vi "Mult-Plex Switch POC.Async.vi"(10 "Parameters":variant, 11 "Process":refnum<class "Process.lvclass">) -> ()   [LabVIEW 2021, in "Software Multi-Plex Engine.lvlib"]
uses:
  Software Multi-Plex Engine.lvlib
  <vilib>/NI/NIVS Inline Async API/_VS Inline Async API/Process/Process.lvclass
  <vilib>/NI/NIVS Inline Async API/_VS Inline Async API/Process/Process.lvclass/Process.ctl
  Shared/Compiled.Settings.ctl
  <vilib>/NI/NIVS Inline Async API/_Data Access Engine/Access Type Classes/Read/Read.lvclass/Read.ctl
  <vilib>/NI/NIVS Inline Async API/_Data Access Engine/Access Type Classes/Write/Write.lvclass/Write.ctl
  <vilib>/NI/NIVS Inline Async API/_Data Access Engine/Data Access Engine/Methods/Read.Data.Detect.vi
  <vilib>/NI/NIVS Inline Async API/_Data Access Engine/Data Access Engine/Methods/Write.Data.vi
  <vilib>/NI/NIVS Inline Async API/_VS Inline Async API/Process/Data Member Access/Read Data Access.vi
  <vilib>/NI/NIVS Inline Async API/_VS Inline Async API/Error Handling Process/SubVIs/Error.ConvertArray.vi
  <vilib>/NI/NIVS Inline Async API/_Data Access Engine/Access Type Classes/Read/Read.ProcessData.Detect.vi
  <vilib>/NI/NIVS Inline Async API/_Data Access Engine/Access Type Classes/Write/Write.ProcessData.vi
  <vilib>/NI/NIVS Inline Async API/_Data Access Engine/Access Type Classes/Write/Write.Buffer.vi
  <vilib>/NI/NIVS Inline Async API/_Data Access Engine/Access Type Classes/Write/Write.Commit.vi
  <vilib>/NI/NIVS Inline Async API/_Data Access Engine/Data Access Engine/Methods/Read.Lookup.vi
  <vilib>/NI/NIVS Inline Async API/_Data Access Engine/Data Access Engine/Methods/Write.Lookup.vi
  <vilib>/NI/NIVS Inline Async API/_Data Access Engine/Data Access Engine/Data Access Engine.lvclass
  Shared/Software Multi-Plex Shared.lvlib
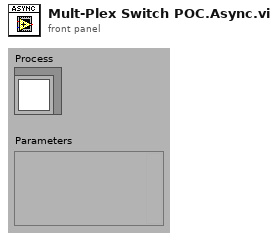
[diagram p1: front panel]
types:
  T1 = typedef "Software Multi-Plex Shared.lvlib/Compiled.Settings.ctl" = cluster{"Name":string, "Number of Channels":i32, "Inputs per Channel":i32, "Global Selector":bool}
  T2 = typedef "Data Access Engine.lvlib/Data Access Engine.lvclass/Read.DVR.ctl" = refnum<data-value>
  T3 = typedef "Data Access Engine.lvlib/Data Access Engine.lvclass/Write.DVR.ctl" = refnum<data-value>
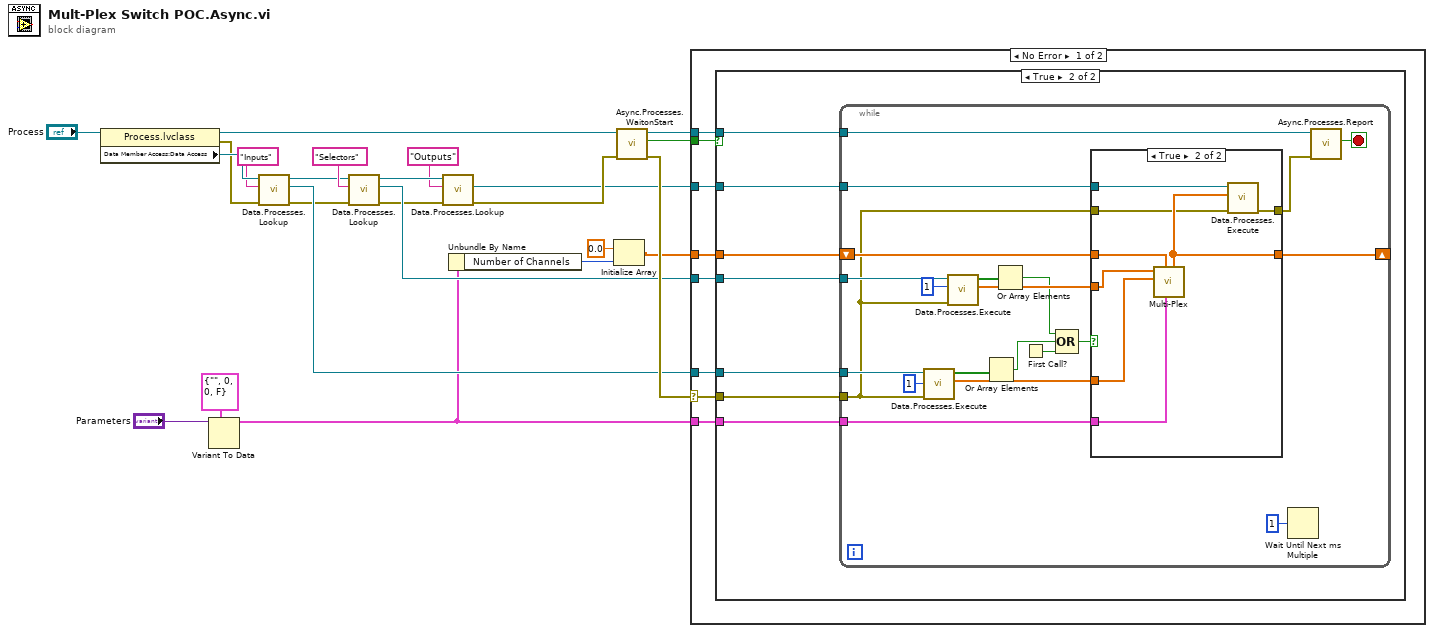
[diagram p0: block diagram]
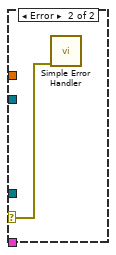
[diagram p4: hidden frame]
diagram:
  n1 = property class="Process.lvclass"(reference="Process") -> (reference out=w20:refnum<class "Process.lvclass">, error out=w13:errorcluster, "Data Member Access:Data Access"=w14:refnum<class "Data Access Engine.lvclass">)  [unwired: 1 in]
  n2 = Variant To Data(type=T1 {"Name"="", "Number of Channels"=0, "Inputs per Channel"=0, "Global Selector"=FALSE} ("Compiled.Settings"), Variant="Parameters") -> (data=w2:T1)  [unwired: 1 in, 1 out]
  n3 = call-poly <vilib>:"Data.Processes.Lookup.vi"("error in (no error)"=w13, "Name"="Inputs", "Data Access API in"=w14) -> ("error out"=w6:errorcluster, "Ref"=w12:T2, "Data Access API out"=w5:refnum<class "Data Access Engine.lvclass">)  [unwired: 5 in, 1 out]
  n4 = call-poly <vilib>:"Data.Processes.Lookup.vi"("error in (no error)"=w6, "Name"="Selectors", "Data Access API in"=w5) -> ("error out"=w9:errorcluster, "Ref"=w16:T2, "Data Access API out"=w19:refnum<class "Data Access Engine.lvclass">)  [unwired: 5 in, 1 out]
  n5 = call-poly <vilib>:"Data.Processes.Lookup.vi"("error in (no error)"=w9, "Name"="Outputs", "Data Access API in"=w19) -> ("error out"=w17:errorcluster, "Ref"=w15:T3)  [unwired: 5 in, 2 out]
  n6 = Unbundle By Name(w2) -> ("Number of Channels"=w1:i32)
  n7 = Initialize Array(0.0 ("element"), w1) -> (w3:dbl[])
  n8 = call <vilib>:"Async.Processes.WaitonStart.vi"("error in (no error)"=w17, "Process"=w20) -> ("error out"=w22:errorcluster, "Execute"=w24:bool, "Process out"=w23:refnum<class "Process.lvclass">)  [unwired: 7 in]
  n9 = case shown="No Error" w22 {
    selector: w22 -> [w30 w71]
    tunnel: w24 -> [w32 _]
    tunnel: w23 -> [w31 _]
    tunnel: w16 -> [w29 _]
    tunnel: w15 -> [w28 _]
    tunnel: w12 -> [w27 _]
    tunnel: w2 -> [w26 _]
    tunnel: w3 -> [w25 _]
    frame No Error {
      n10 = case shown="True" w32 {
        tunnel: w30 -> [_ w38]
        tunnel: w31 -> [_ w39]
        tunnel: w29 -> [_ w37]
        tunnel: w28 -> [_ w36]
        tunnel: w27 -> [_ w35]
        tunnel: w26 -> [_ w34]
        tunnel: w25 -> [_ w33]
        frame False {
        }
        frame True {
          n11 = while {
            tunnel: w38 -> [w40]
            tunnel: w39 -> [w60]
            tunnel: w37 -> [w58]
            tunnel: w36 -> [w57]
            tunnel: w35 -> [w50]
            tunnel: w34 -> [w44]
            shift-right: [w43] -> _
            shift-left: w33 -> [w42]
            stop <- w59 stop-if-true
            n12 = call-poly <vilib>:"Data.Processes.Execute.vi"("error in (no error)"=w40, "timeout ms"=1, "Ref"=w50) -> ("Values"=w49:dbl[], "Detect?"=w51:bool[])  [unwired: 5 in, 2 out]
            n13 = call-poly <vilib>:"Data.Processes.Execute.vi"("error in (no error)"=w40, "timeout ms"=1, "Ref"=w58) -> ("Values"=w56:dbl[], "Detect?"=w55:bool[])  [unwired: 5 in, 2 out]
            n14 = Or Array Elements(Boolean array=w51) -> (logical OR=w46:bool)
            n15 = Or Array Elements(Boolean array=w55) -> (logical OR=w53:bool)
            n16 = First Call?() -> (First Call?: T/F=w45:bool)
            n17 = Compound Arithmetic op=OR(w53, w46, w45) -> (w54:bool)
            n18 = case shown="True" w54 {
              tunnel: w57 -> [_ w70]
              tunnel: w56 -> [_ w69]
              tunnel: w49 -> [_ w68]
              tunnel: w44 -> [_ w67]
              tunnel: [w62 w65] -> w43
              tunnel: [w61 w66] -> w41
              tunnel: w42 -> [w62 w64]
              tunnel: w40 -> [w61 w63]
              frame False {
              }
              frame True {
                n19 = call "Multi-Plex.vi"("Settings"=w67, "Prev Outputs"=w64, "Inputs"=w68, "Control"=w69) -> ("Outputs"=w65:dbl[])  [unwired: 7 in]
                n20 = call-poly <vilib>:"Data.Processes.Execute.vi"("error in (no error)"=w63, "Values"=w65, "Ref"=w70) -> ("error out"=w66:errorcluster)  [unwired: 8 in]
              }
            }
            n21 = Wait Until Next ms Multiple(millisecond multiple=u32 1) -> ()  [unwired: 1 out]
            n22 = call <vilib>:"Async.Processes.Report.vi"("Error"=w41, "Process in"=w60) -> ("Stop"=w59:bool)  [unwired: 8 in, 1 out]
          }
        }
      }
    }
    frame Error {
      n23 = call <vilib>:"Simple Error Handler.vi"("error in (no error)"=w71) -> ()  [unwired: 4 in, 5 out]
    }
  }
